vi "subpanelStopUI.vi"(8 "error in (no error)":errorcluster, 10 "UI VI*":refnum<vi>, 11 "xceDataNode in":refnum<class "xceDataNode.lvclass">) -> (0 "error out":errorcluster, 3 "xceDataNode out":refnum<class "xceDataNode.lvclass">)   [LabVIEW 2013, in "xceDataNode.lvclass"]
doc: "Community access for the method StopUI method. Used to give access to the xceSubpanel class."
uses:
  xceDataNode.lvclass
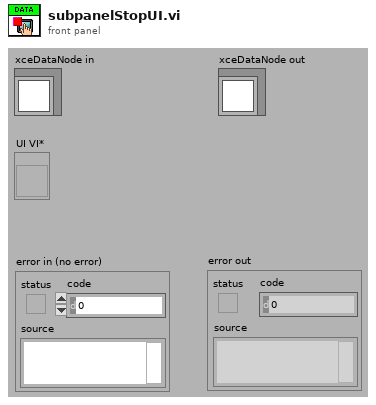
[diagram p1: front panel]
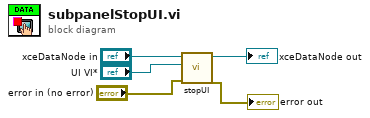
[diagram p0: block diagram]
diagram:
  n1 = call-dynamic "stopUI.vi"("error in (no error)"="error in (no error)", "UI VI*"="UI VI*", "xceDataNode in"="xceDataNode in") -> ("error out"=→"error out":errorcluster, "xceDataNode out"=→"xceDataNode out":refnum<class "xceDataNode.lvclass">)  [unwired: 7 in]
